vi "get_cmds.vi"(11 "Joysticks":T4) -> (3 "Commands":T1)   [LabVIEW 2012]
uses:
  <vilib>/Rock Robotics/WPI/Joystick/WPI_JoystickButtonState.ctl
  util/Commands.ctl
  climber/climber_cmds.ctl
panel:
  in  "Commands 2":T1
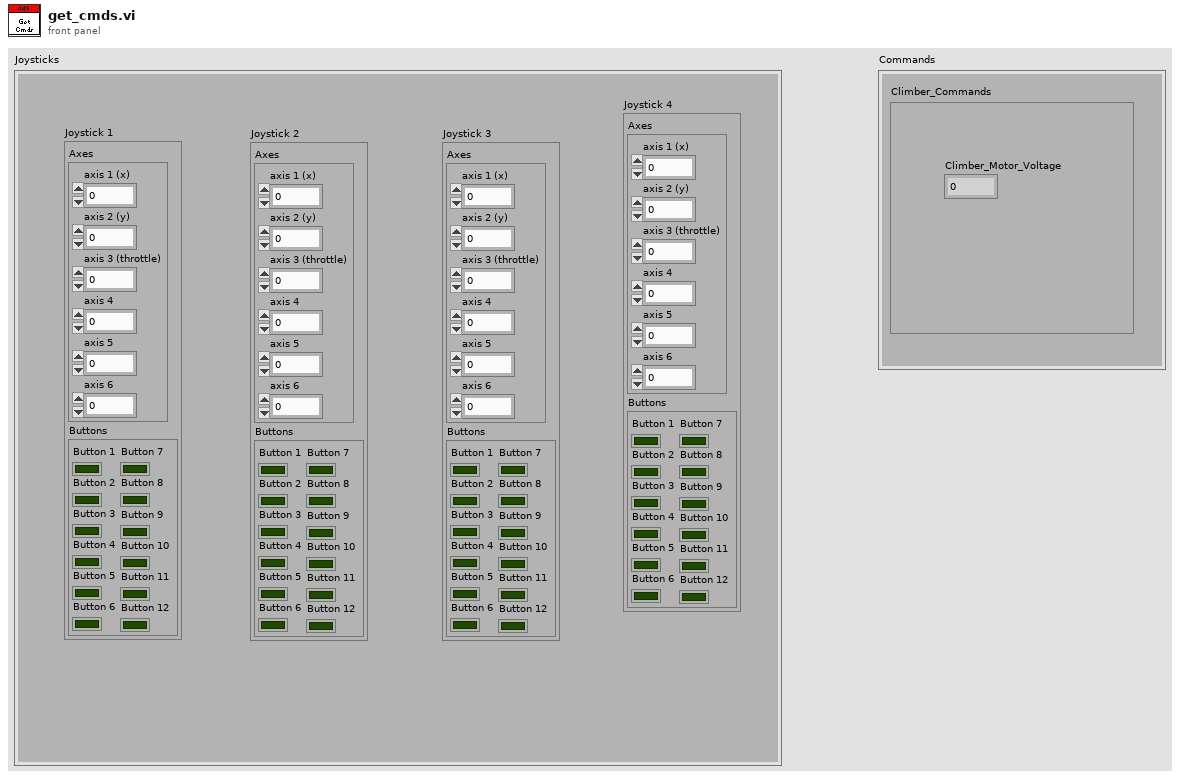
[diagram p1: front panel]
types:
  T1 = typedef "Commands.ctl" = cluster{"Climber_Commands":T2}
  T2 = typedef "climber_cmds.ctl" = cluster{"Climber_Motor_Voltage":dbl}
  T3 = typedef "WPI_JoystickButtonState.ctl" = cluster{"Button 1":bool, "Button 2":bool, "Button 3":bool, "Button 4":bool, "Button 5":bool, "Button 6":bool, "Button 7":bool, "Button 8":bool, "Button 9":bool, "Button 10":bool, "Button 11":bool, "Button 12":bool}
  T4 = cluster{"Joystick 1":cluster{"Axes":cluster{"axis 1 (x)":dbl, "axis 2 (y)":dbl, "axis 3 (throttle)":dbl, "axis 4":dbl, "axis 5":dbl, "axis 6":dbl}, "Buttons":T3}, "Joystick 2":cluster{"Axes":cluster{"axis 1 (x)":dbl, "axis 2 (y)":dbl, "axis 3 (throttle)":dbl, "axis 4":dbl, "axis 5":dbl, "axis 6":dbl}, "Buttons":T3}, "Joystick 3":cluster{"Axes":cluster{"axis 1 (x)":dbl, "axis 2 (y)":dbl, "axis 3 (throttle)":dbl, "axis 4":dbl, "axis 5":dbl, "axis 6":dbl}, "Buttons":T3}, "Joystick 4":cluster{"Axes":cluster{"axis 1 (x)":dbl, "axis 2 (y)":dbl, "axis 3 (throttle)":dbl, "axis 4":dbl, "axis 5":dbl, "axis 6":dbl}, "Buttons":T3}}
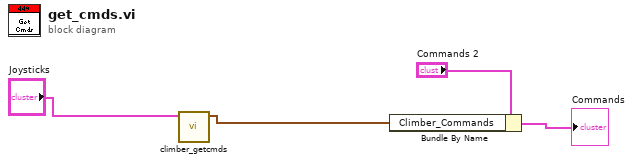
[diagram p0: block diagram]
diagram:
  n1 = call "climber_getcmds.vi"("Joysticks"="Joysticks") -> ("Climber_Commands"=w1:T2)  [unwired: 10 in]
  n2 = Bundle By Name(cluster="Commands 2", "Climber_Commands"=w1) -> (→"Commands":T1)
